vi "Read Line Rate - With One Method - Returns Total Value.vi"() -> ()   [LabVIEW 2017, in "Cobertura.Tests.lvlib" / "Package.lvlib"]
uses:
  Package.lvlib
  Cobertura/Package/Package.lvclass/Package.ctl
  Cobertura/Package/Read Line Rate.vi
  <vilib>/PNR/Transparent Assertions/Transparent Assertions/Transparent Assertions.lvlib
  Cobertura/Class/Class.lvclass
  Cobertura/Method/Method.lvclass
  Cobertura/Package/Package.lvclass
panel:
  out "error out":errorcluster
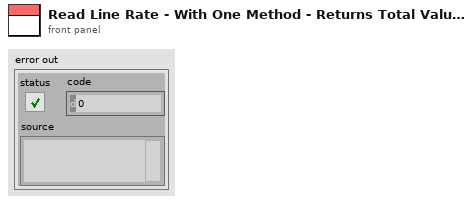
[diagram p1: front panel]
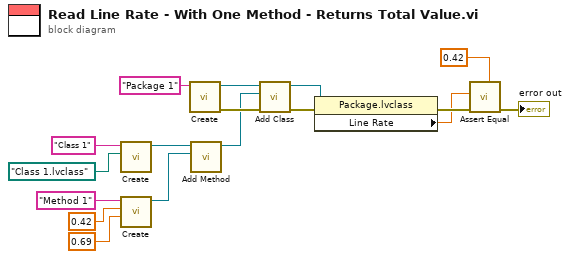
[diagram p0: block diagram]
diagram:
  n1 = call "Create.vi"("Filename"=path "Class 1.lvclass", "Name"="Class 1") -> ("Class"=w14:refnum<class "Class.lvclass">)  [unwired: 8 in, 1 out]
  n2 = call "Create.vi"("Branch Rate"=0.69, "Line Rate"=0.42, "Name"="Method 1") -> ("Method"=w10:refnum<class "Method.lvclass">)  [unwired: 7 in, 1 out]
  n3 = call "Create.vi"("Name"="Package 1") -> ("error out"=w7:errorcluster, "Package"=w4:refnum<class "Package.lvclass">)  [unwired: 9 in]
  n4 = call "Add Method.vi"("Method"=w10, "Class in"=w14) -> ("Class out"=w2:refnum<class "Class.lvclass">)  [unwired: 8 in, 1 out]
  n5 = call "Add Class.vi"("error in (no error)"=w7, "Class"=w2, "Package in"=w4) -> ("error out"=w6:errorcluster, "Package out"=w3:refnum<class "Package.lvclass">)  [unwired: 7 in]
  n6 = property class="Package.lvclass"(reference=w3, error in=w6) -> (error out=w16:errorcluster, "Line Rate"=w9:dbl)  [unwired: 1 out]
  n7 = call <vilib>:"Assert Equal.vi"("Expected"=0.42 ("Branch Rate"), "error in (no error)"=w16, "Actual"=w9) -> ("error out"=→"error out":errorcluster)  [unwired: 8 in]
